vi "Pos ctrl window-Initialise globals.vi"   [LabVIEW 2017]
uses:
  Globals/Pos ctrl window globals.vi
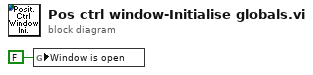
[diagram p0: block diagram]
diagram:
  n1 = global write "Pos ctrl window globals.vi" "Window is open"(FALSE ("Bring to front")) -> ()
